vi "ReadWrite Top Level.vi"(6 "Iteration":i32, 7 "Mode":T23, 8 "error in (no error)":errorcluster, 9 "Iteration Duration":i64, 11 "RT Data in":T1 {"SEA9811_RT_data"."Tx"."Tx Refs (Data,Trig)"."Data Reference" format="%.0x"; "Label Transfer Config"."Block Data Refs"."Data Reference" format="%.0x"; "Status Config"."HWOut Dur Ref" format="%.0x"; "Status Config"."HWIn Dur Ref" format="%.0x"; "Status Config"."Error Data Ref" format="%.0x"; "HWOutput Channels"."Labels Settings"."Label" format="%.0o"; "HWInput Channels"."Labels Settings"."Label" format="%.0o"}) -> (0 "error out":errorcluster, 3 "RT Data out":T1 {"SEA9811_RT_data"."Tx"."Tx Refs (Data,Trig)"."Data Reference" format="%.0x"; "Label Transfer Config"."Block Data Refs"."Data Reference" format="%.0x"; "Status Config"."HWOut Dur Ref" format="%.0x"; "Status Config"."HWIn Dur Ref" format="%.0x"; "Status Config"."Error Data Ref" format="%.0x"; "HWOutput Channels"."Labels Settings"."Label" format="%.0o"; "HWInput Channels"."Labels Settings"."Label" format="%.0o"})   [LabVIEW 2012, in "AIT 429 Engine.lvlib"]
uses:
  AIT 429 Engine.lvlib
  RT Controls/ReadWrite Selector.ctl
  RT Controls/RT Data.ctl
  <userlib>/_FPGA Interface Advanced Tools/FPGA Interface Base/FPGA Interface Base.lvclass
  RT Controls/RT HW Channel.ctl
  RT Controls/RT Label Settings.ctl
  Shared/Controls and Global/Label.ctl
  Shared/Controls and Global/transferPeriod.ctl
  RT Controls/Driver Data.ctl
  RT Controls/RT Word Settings.ctl
  <vilib>/NI Veristand/Custom Device API/Block Data Reference.ctl
  <vilib>/NI Veristand/Custom Device API/Data Reference.ctl
  RT Controls/RT Param Setting.ctl
  Shared/Controls and Global/Start Bit.ctl
  Shared/Controls and Global/Number of Bits.ctl
  Shared/Controls and Global/TransferType.ctl
  RT Controls/Error Qs.ctl
  RT Controls/Status Channels Config.ctl
  RT Controls/FIFO.ctl
  RT Controls/Label Transfer Config.ctl
  SEA 9811 FPGA driver/RT/Typdefs/SEA9811_RT_data_cluster.ctl
  SEA 9811 FPGA driver/RT/Typdefs/FPGA ref.ctl
  SEA 9811 FPGA driver/RT/Typdefs/channel.ctl
  SEA 9811 FPGA driver/RT/Typdefs/received word.ctl
  SEA 9811 FPGA driver/RT/Typdefs/SEA9811_FPGA_FP_Addresses.ctl
  <vilib>/NI Veristand/Custom Device API/NI VeriStand - Get Channel Values by Block Data Reference.vi
  <vilib>/NI Veristand/Custom Device API/NI VeriStand - Set Channel Value by Data Reference.vi
  <vilib>/NI Veristand/Custom Device API/Global Data Refs.vi
  <vilib>/NI Veristand/Custom Device API/Custom Device API.lvlib
  Shared/ARINC 429 Shared.lvlib
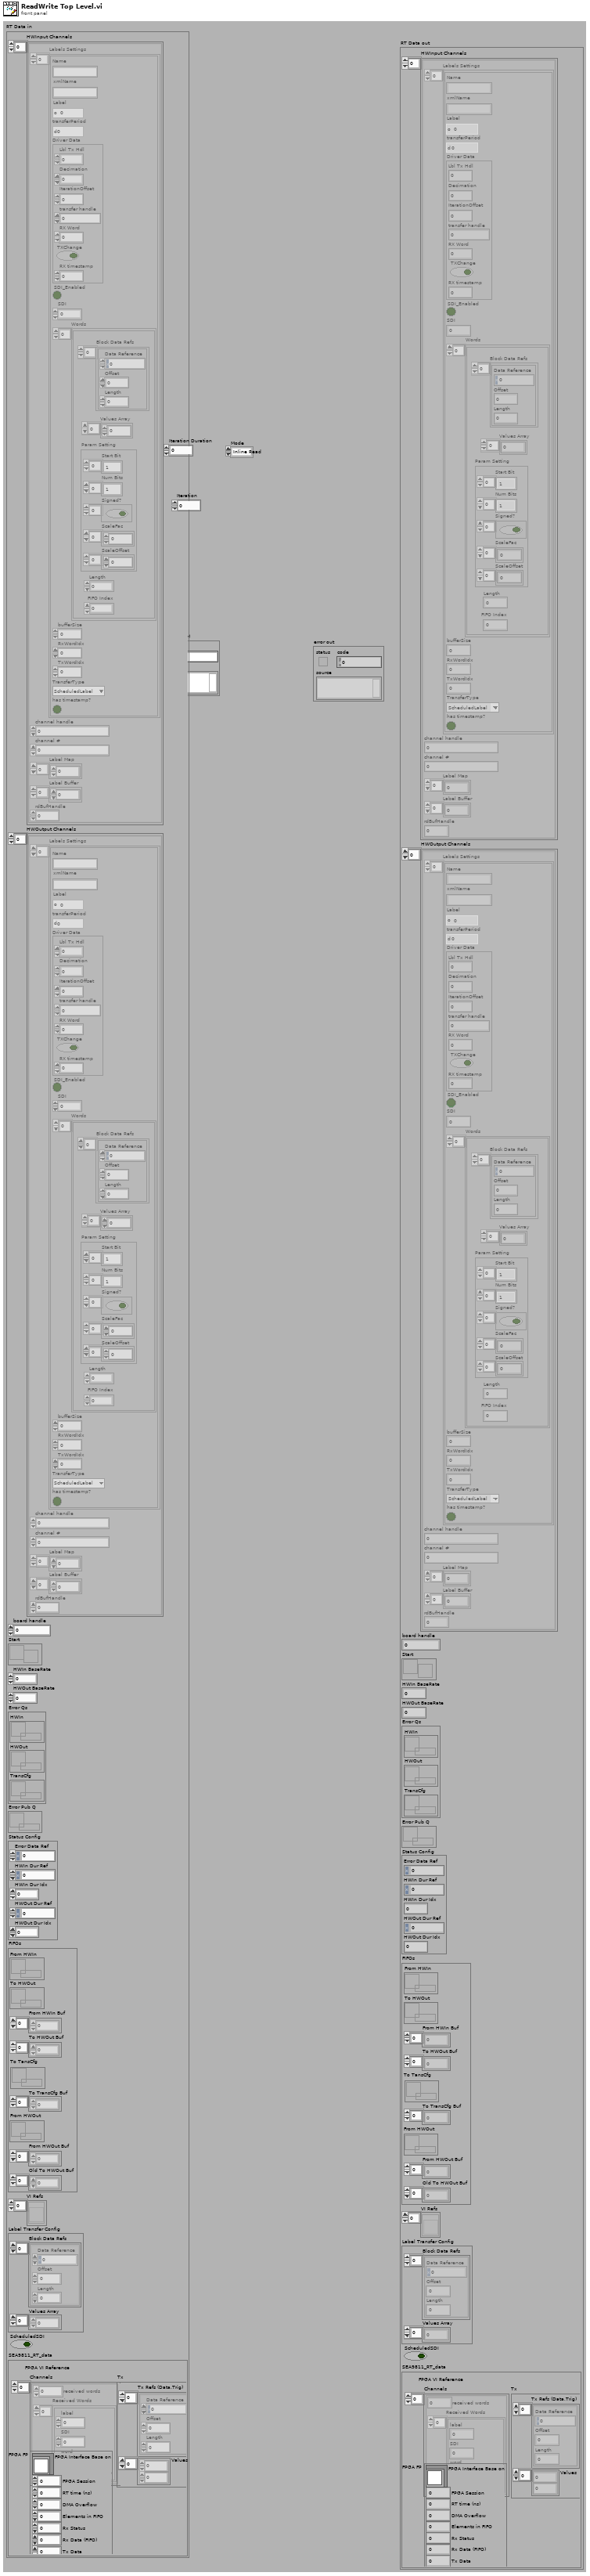
[diagram p1: front panel]
types:
  T1 = typedef "AIT 429 Engine.lvlib/RT Data.ctl" = cluster{"HWInput Channels":T2[], "HWOutput Channels":T2[], "board handle":u32, "Start":refnum<notifier>, "HWIn BaseRate":i64, "HWOut BaseRate":i64, "Error Qs":T14, "Error Pub Q":refnum<queue>, "Status Config":T15, "FIFOs":T16, "VI Refs":refnum<vi>[], "Label Transfer Config":T17, "ScheduledSDI":bool, "SEA9811_RT_data":T18}
  T2 = typedef "AIT 429 Engine.lvlib/RT HW Channel.ctl" = cluster{"Labels Settings":T3[], "channel handle":u32, "channel #":u16, "Label Map":i32[], "Label Buffer":u32[], "rdBufHandle":u32}
  T3 = typedef "AIT 429 Engine.lvlib/RT Label Settings.ctl" = cluster{"Name":string, "xmlName":string, "Label":T4, "transferPeriod":T5, "Driver Data":T6, "SDI_Enabled":bool, "SDI":u8, "Words":T7[], "bufferSize":u32, "RxWordIdx":i32, "TxWordIdx":i32, "TransferType":T13, "has timestamp?":bool}
  T4 = typedef "ARINC 429 Shared.lvlib/Label.ctl" = u8
  T5 = typedef "ARINC 429 Shared.lvlib/transferPeriod.ctl" = u32
  T6 = typedef "AIT 429 Engine.lvlib/Driver Data.ctl" = cluster{"Lbl Tx Hdl":u32, "Decimation":i32, "IterationOffset":i32, "transfer handle":u32, "RX Word":u32, "TXChange":bool, "RX timestamp":dbl}
  T7 = typedef "AIT 429 Engine.lvlib/RT Word Settings.ctl" = cluster{"Block Data Refs":T8[], "Values Array":dbl[], "Length":i32, "FIFO Index":i32, "Param Setting":T10}
  T8 = typedef "Custom Device API.lvlib/Block Data Reference.ctl" = cluster{"Data Reference":T9, "Offset":i32, "Length":i32}
  T9 = typedef "Custom Device API.lvlib/Data Reference.ctl" = i32
  T10 = typedef "AIT 429 Engine.lvlib/RT Param Setting.ctl" = cluster{"Start Bit":T11[], "Num Bits":T12[], "Signed?":bool[], "ScaleFac":dbl[], "ScaleOffset":dbl[]}
  T11 = typedef "ARINC 429 Shared.lvlib/Start Bit.ctl" = i32
  T12 = typedef "ARINC 429 Shared.lvlib/Number of Bits.ctl" = i32
  T13 = typedef "ARINC 429 Shared.lvlib/TransferType.ctl" = enum16{"ScheduledLabel", "Acyclic", "Block", "Strobe"}
  T14 = typedef "AIT 429 Engine.lvlib/Error Qs.ctl" = cluster{"HWIn":refnum<queue>, "HWOut":refnum<queue>, "TransCfg":refnum<queue>}
  T15 = typedef "AIT 429 Engine.lvlib/Status Channels Config.ctl" = cluster{"Error Data Ref":T9, "HWIn Dur Ref":T9, "HWIn Dur Idx":i32, "HWOut Dur Ref":T9, "HWOut Dur Idx":i32}
  T16 = typedef "AIT 429 Engine.lvlib/FIFO.ctl" = cluster{"From HWIn":refnum<k33>, "To HWOut":refnum<k33>, "From HWIn Buf":dbl[], "To HWOut Buf":dbl[], "To TansCfg":refnum<k33>, "To TransCfg Buf":dbl[], "From HWOut":refnum<k33>, "From HWOut Buf":dbl[], "Old To HWOut Buf":dbl[]}
  T17 = typedef "AIT 429 Engine.lvlib/Label Transfer Config.ctl" = cluster{"Block Data Refs":T8[], "Values Array":dbl[]}
  T18 = typedef "SEA9811_RT_data_cluster.ctl" = cluster{"FPGA VI Reference":T19, "Channels":T20[], "FPGA FP":T22, "Tx":cluster{"Tx Refs (Data,Trig)":T8[], "Values":dbl[]}}
  T19 = typedef "FPGA ref.ctl" = refnum<k20>
  T20 = typedef "channel.ctl" = cluster{"received words":u32, "Received Words":T21[]}
  T21 = typedef "received word.ctl" = cluster{"label":u8, "SDI":u8, "word":u32, "timestamp":dbl}
  T22 = typedef "SEA9811_FPGA_FP_Addresses.ctl" = cluster{"FPGA Interface Base on":refnum<class "FPGA Interface Base.lvclass">, "FPGA Session":u32, "RT time (ns)":u32, "DMA Overflow":u32, "Elements in FIFO":u32, "Rx Status":u32, "Rx Data (FIFO)":u32, "Tx Data":u32, "Transmit Data":u32}
  T23 = typedef "AIT 429 Engine.lvlib/ReadWrite Selector.ctl" = enum16{"Inline Read", "Inline Write", "Async HWIn", "Async HWOut"}
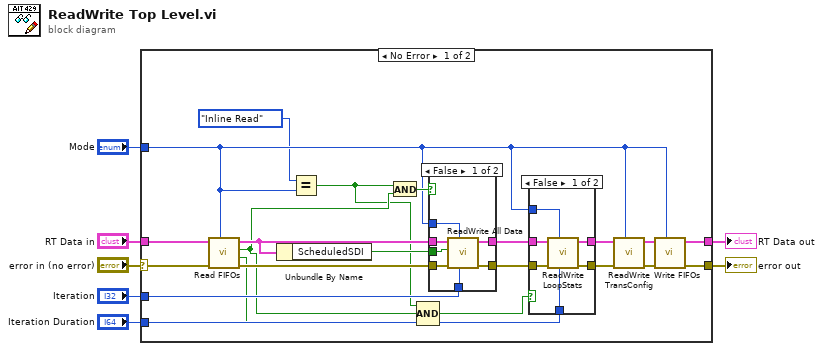
[diagram p0: block diagram]
diagram:
  n1 = case shown="No Error" "error in (no error)" {
    selector: "error in (no error)" -> [w23 w48]
    tunnel: "RT Data in" -> [w29 w47]
    tunnel: [w28 w47] -> w1
    tunnel: [w27 w48] -> w7
    tunnel: "Mode" -> [w13 _]
    tunnel: "Iteration" -> [w19 _]
    tunnel: "Iteration Duration" -> [w11 _]
    frame No Error {
      n2 = call "Read FIFOs.vi"("Mode"=w13, "error in (no error)"=w23, "RT Data in"=w29) -> ("error out"=w26:errorcluster, "Empty From HWOut"=w8:bool, "Empty From HWIn"=w18:bool, "RT Data out"=w25:T1)  [unwired: 5 in]
      n3 = Unbundle By Name(w25) -> ("ScheduledSDI"=w20:bool)
      n4 = Equal?(x=ReadWrite_Selector."Inline Read", y=w13) -> (x = y?=w12:bool)
      n5 = And(x=w12, y=w18) -> (x .and. y?=w24:bool)
      n6 = Compound Arithmetic op=AND(w12, w18, w8) -> (w9:bool)
      n7 = case shown="False" w24 {
        tunnel: w26 -> [w44 w46]
        tunnel: [w38 w46] -> w17
        tunnel: [w39 w45] -> w16
        tunnel: w25 -> [w43 w45]
        tunnel: w13 -> [w41 _]
        tunnel: w19 -> [w42 _]
        tunnel: w20 -> [w40 _]
        frame False {
          n8 = call "ReadWrite All Data.vi"("Iteration"=w42, "Mode"=w41, "error in (no error)"=w44, "ScheduledSDI"=w40, "RT Data in"=w43) -> ("error out"=w38:errorcluster, "RT Data out"=w39:T1)  [unwired: 5 in]
        }
        frame True {
        }
      }
      n9 = case shown="False" w9 {
        tunnel: w17 -> [w35 w37]
        tunnel: w16 -> [w34 w36]
        tunnel: [w33 w36] -> w15
        tunnel: [w32 w37] -> w14
        tunnel: w13 -> [w31 _]
        tunnel: w11 -> [w30 _]
        frame False {
          n10 = call "ReadWrite LoopStats.vi"("Iteration Duration"=w30, "Mode"=w31, "error in (no error)"=w35, "RT Data in"=w34) -> ("error out"=w32:errorcluster, "RT Data out"=w33:T1)  [unwired: 6 in]
        }
        frame True {
        }
      }
      n11 = call "ReadWrite TransConfig.vi"("Mode"=w13, "error in (no error)"=w14, "RT Data in"=w15) -> ("error out"=w21:errorcluster, "RT Data out"=w22:T1)  [unwired: 7 in]
      n12 = call "Write FIFOs.vi"("Mode"=w13, "error in (no error)"=w21, "RT Data in"=w22) -> ("error out"=w27:errorcluster, "RT Data out"=w28:T1)  [unwired: 7 in]
    }
    frame Error {
    }
  }
  "error out" <- w7
  "RT Data out" <- w1
